vi "Real-Time-UDP.vi"() -> ()   [LabVIEW 2016]
uses:
  <vilib>/userdefined/High Color/IMAQdx.ctl
  <vilib>/FPGAPlugInAG/roboRIO/niLvFpga_Open_roboRIO.vi
  <vilib>/rvi/interface/common/dynamic/niFpgaDynamicAddResources.vi
  <vilib>/FPGAPlugInAG/Dynamic/niLvFpga_Download_Dynamic.vi
  <vilib>/FPGAPlugInAG/Dynamic/niLvFpga_Run_Dynamic.vi
  <vilib>/Utility/error.llb/Error Cluster From Error Code.vi
  <vilib>/rvi/errors/niLvFpgaAdjustHostInterfaceError.vi
  <vilib>/rvi/interface/common/niFpgaWaitOnOcc.vi
  <vilib>/vision/EDVR.llb/IMAQ ImageToEDVR 2D U32.vi
  <vilib>/FPGAPlugInAG/Dynamic/niLvFpga_Close_Dynamic.vi
  <vilib>/rvi/interface/nirviOpenFPGA/nirviOpenFPGA.xnode
  FPGA Bitfiles/ImageProcessingw_FPGATarget_ImageProcessing-_HE-F2dzEpTo.lvbitx
  <vilib>/rvi/interface/nirviMethod/nirviMethod.xnode
  <vilib>/rvi/interface/nirviReadWriteControl/nirviReadWriteControl.xnode
  <vilib>/rvi/interface/nirviCloseFPGA/nirviCloseFPGA.xnode
  <vilib>/vision/driver/NI_Vision_Acquisition_Software.lvlib
  <resource>/objmgr/imaqdx.rc
  <vilib>/rvi/interface/Simulation/niFpgaSimulationCallBeginRW.vi
  <vilib>/rvi/errors/niLvFpgaMergeErrorWithErrorCode.vi
  <vilib>/FPGAPlugInAG/Dynamic/niLvFpga_ReadFifo_Dynamic.vi
  <vilib>/FPGAPlugInAG/Dynamic/niLvFpga_ConfigureFifo_Dynamic.vi
  <vilib>/FPGAPlugInAG/Dynamic/niLvFpga_StartFifo_Dynamic.vi
  NiFpgaLv.dll
  <vilib>/FPGAPlugInAG/Dynamic/niLvFpga_WriteFifo_Dynamic.vi
panel:
  out "Image":T1(plugin-control)
  out "Error Out 2":errorcluster
  in  "Stop":bool
  in  "Maximum Pixels per Write":u32=307200
  out "dePixelCount":u32
  out "AllPixelCount":u32
  in  "Camera":T2="cam0"
  # "Overview: Demonstrates how to acquire an image from a camera using the IMAQdx API, transfer the image to a FPGA target for processing, and retrieve the processed image for display or further processing on the host.\nRequirements:\n- LabVIEW FPGA\n- Vision Acquisition Software\n- Vision Development Module\nInstructions:\n1. Select a Camera\n2. Run the VI."
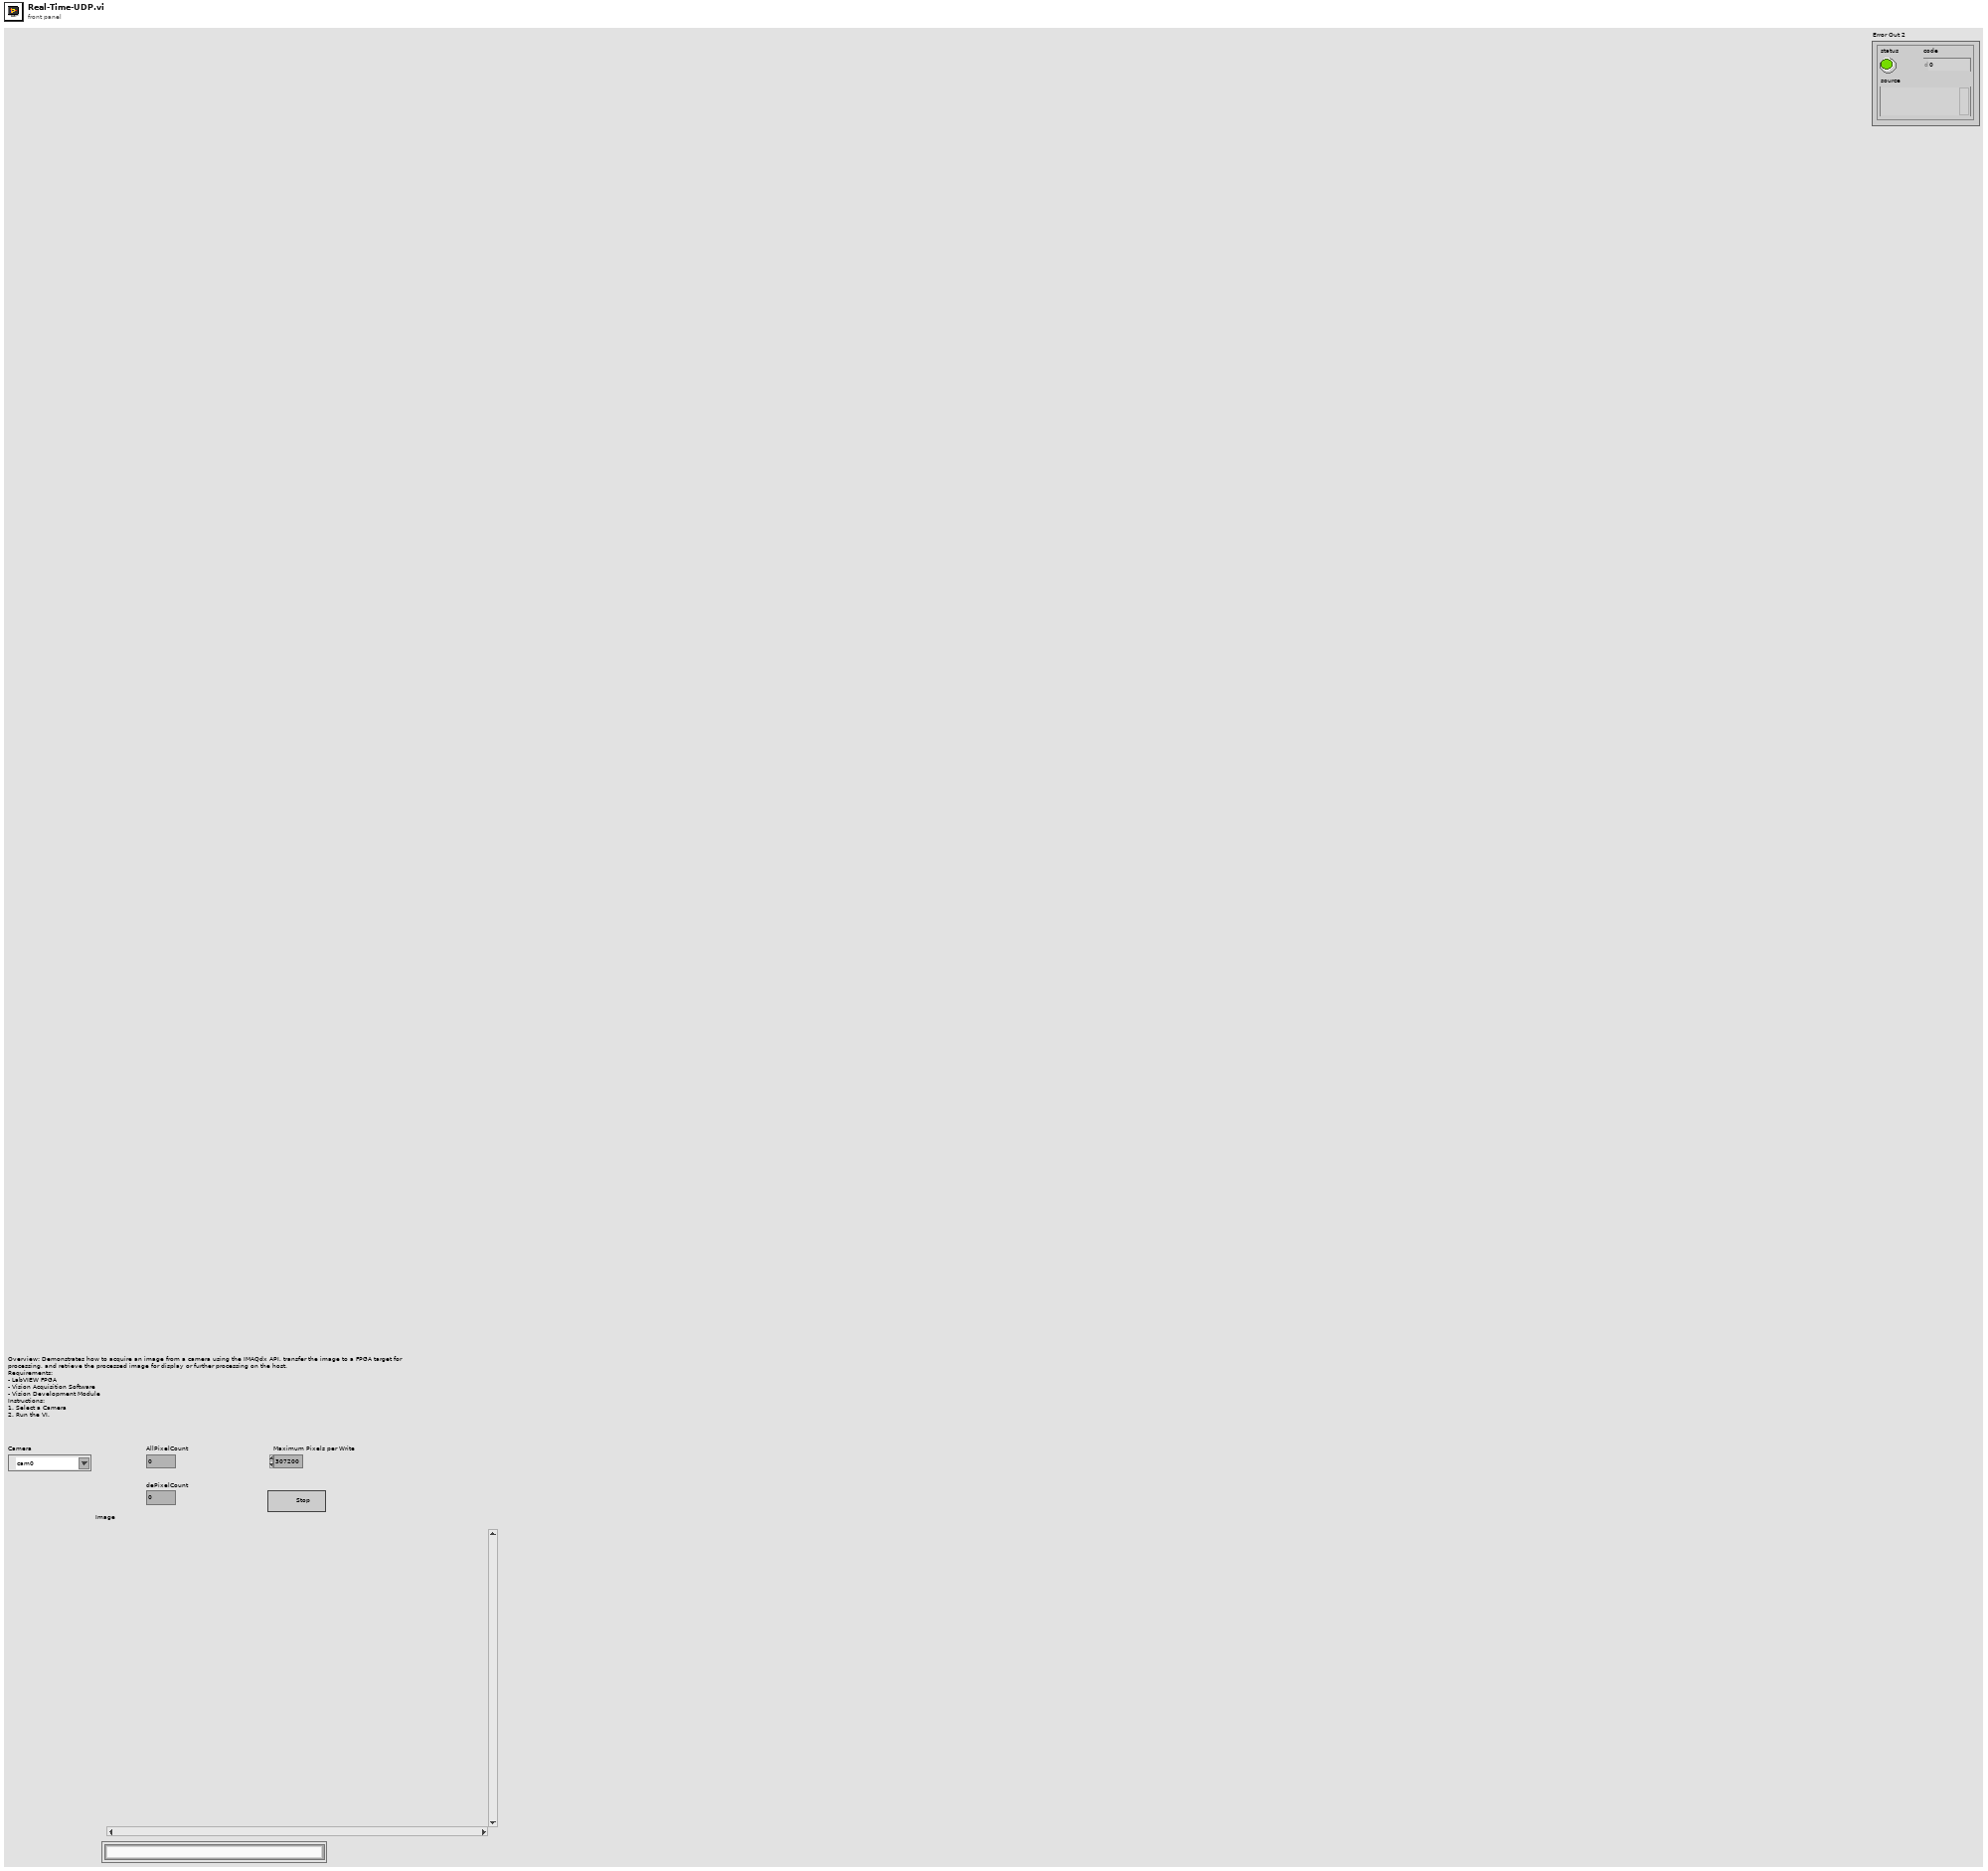
[diagram p1: front panel]
types:
  T1 = typedef "IMAQ Image.ctl" = refnum<image>
  T2 = typedef "IMAQdx.ctl" = refnum<k21>
  T3 = typedef "Image Type" = u32
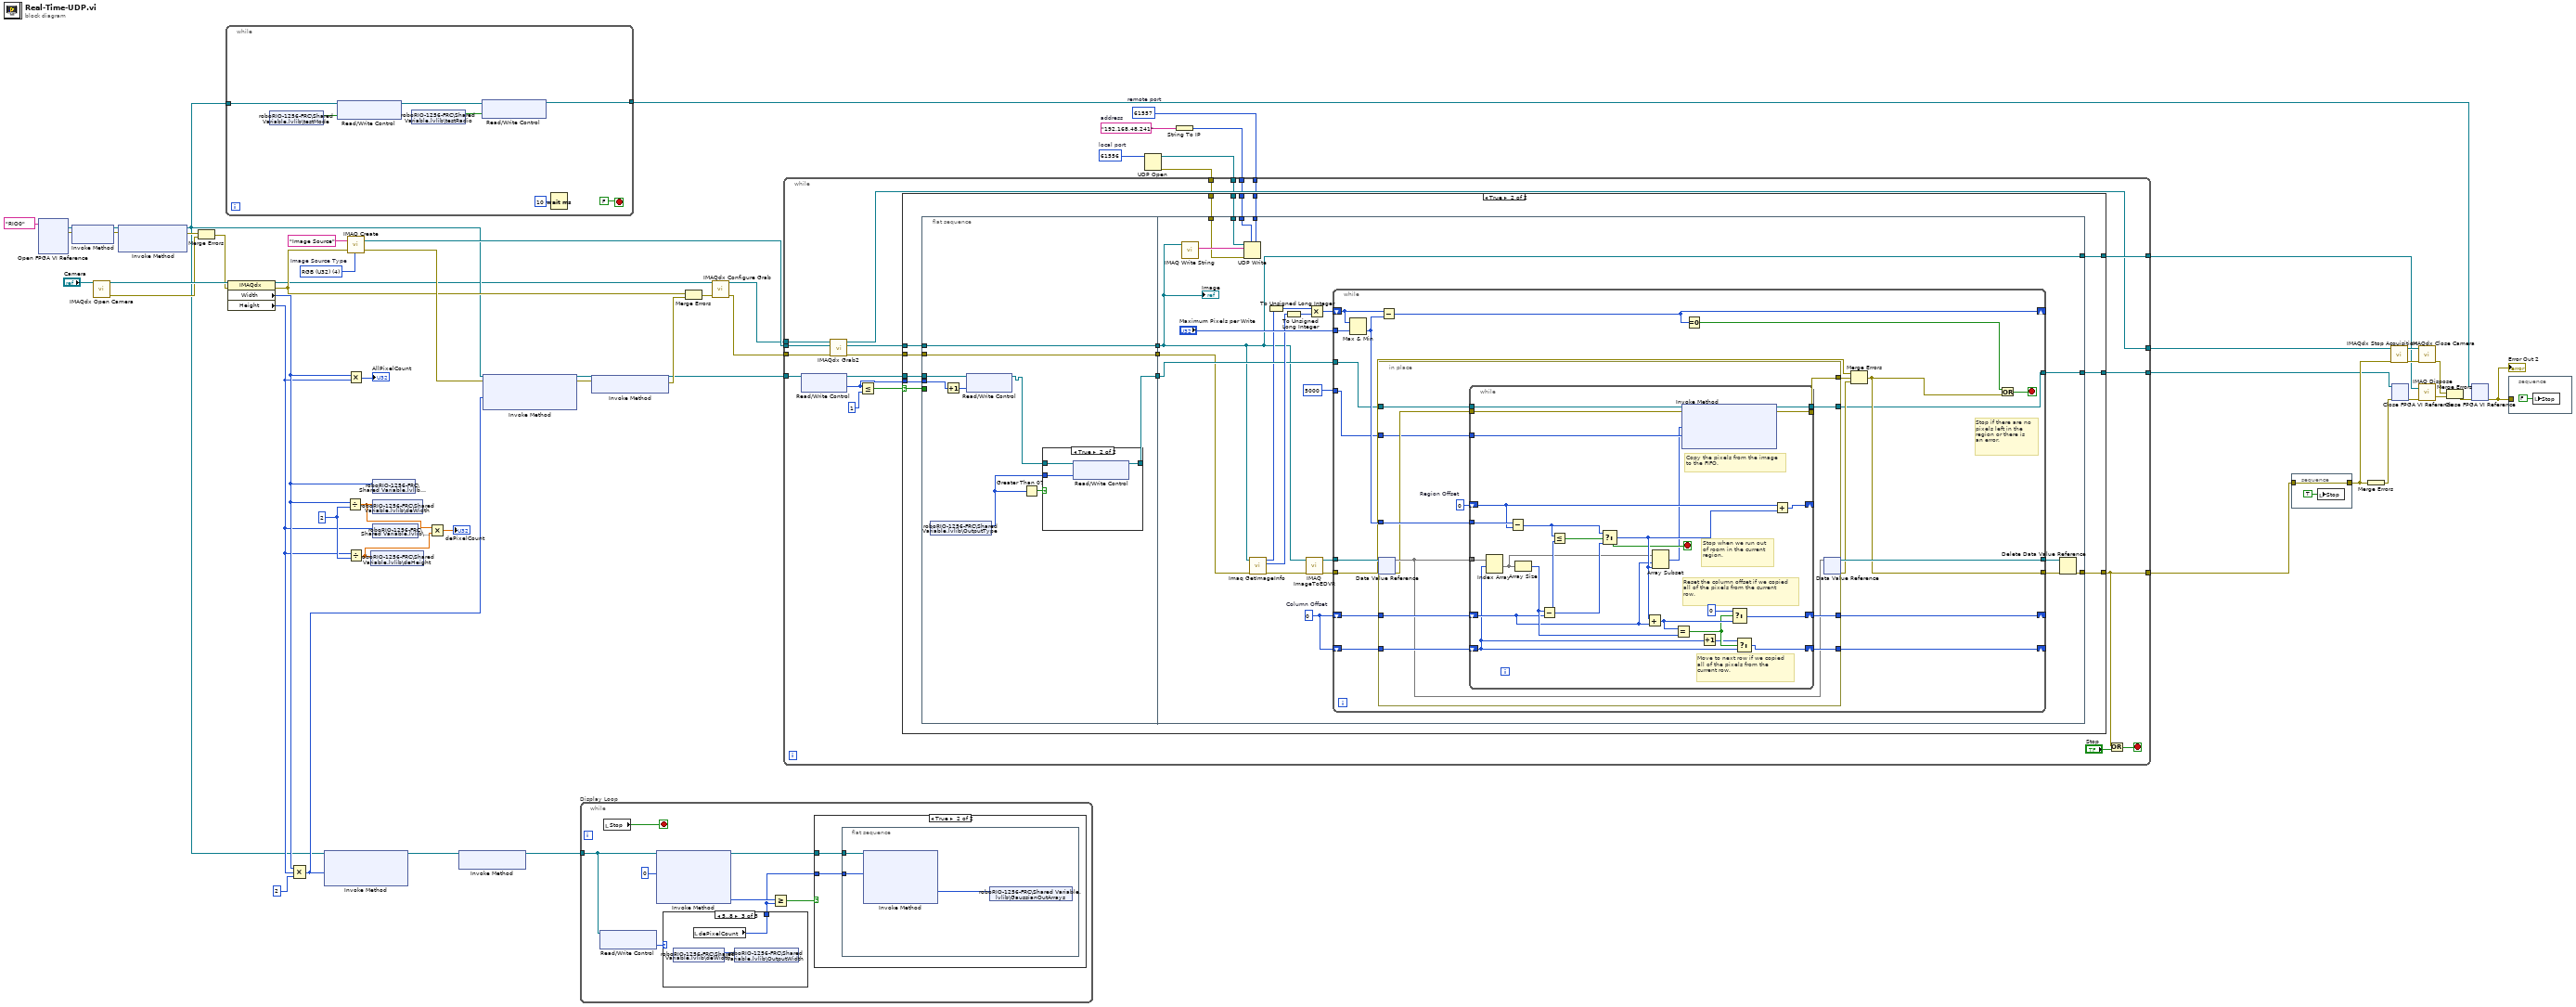
[diagram p0: block diagram]
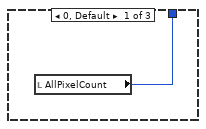
[diagram p4: hidden frame]
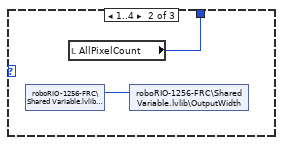
[diagram p5: hidden frame]
diagram:
  w6 = u16 61556  # local port
  w5 = "192.168.48.241"  # address
  w4 = u16 61557  # remote port
  w40 = u32 2 ("y")
  w44 = T3 4 items=["Grayscale (U8)", "Grayscale (I16)", "Grayscale (SGL)", "Complex (CSG)", "RGB (U32)", "HSL (U32)", "RGB (U64)", "Grayscale (U16)"]  # Image Source Type
  n1 = xnode "Open FPGA VI Reference"("resource name"=tag "RIO0") -> ("FPGA VI Reference Out"=w51:refnum<k20>, "error out"=w52:errorcluster)  [unwired: 1 in]
  n2 = xnode "Invoke Method"("FPGA VI Reference In"=w51, "error in"=w52) -> ("FPGA VI Reference Out"=w54:refnum<k20>, "error out"=w53:errorcluster)
  n3 = call <vilib>:"IMAQdx Open Camera.vi"("Session In"="Camera") -> ("error out"=w46:errorcluster, "Session Out"=w47:T2)  [unwired: 9 in]
  n4 = xnode "Invoke Method"("FPGA VI Reference In"=w54, "error in"=w53) -> ("FPGA VI Reference Out"=w11:refnum<k20>, "error out"=w48:errorcluster)  [unwired: 1 in]
  n5 = Merge Errors(w48, w46) -> (w45:errorcluster)
  n6 = while {
    tunnel: w11 -> [w56]
    tunnel: [w57] -> w14
    stop <- FALSE stop-if-true
    n7 = shared-variable "roboRIO-1256-FRC\\Shared Variable.lvlib\\testMode"() -> (w60:bool)  [unwired: 1 in, 1 out]
    n8 = xnode "Read/Write Control"("FPGA VI Reference In"=w56, "Mode LED Status"=w60) -> ("FPGA VI Reference Out"=w59:refnum<k20>)  [unwired: 1 in, 1 out]
    n9 = shared-variable "roboRIO-1256-FRC\\Shared Variable.lvlib\\testRadio"() -> (w58:bool)  [unwired: 1 in, 1 out]
    n10 = xnode "Read/Write Control"("FPGA VI Reference In"=w59, "Radio LED Green"=w58) -> ("FPGA VI Reference Out"=w57:refnum<k20>)  [unwired: 1 in, 1 out]
    n11 = Wait (ms)(milliseconds to wait=u32 10) -> ()  [unwired: 1 out]
  }
  n12 = property class="IMAQdx"(reference=w47, error in=w45) -> (reference out=w10:T2, error out=w29:errorcluster, "Width"=w39:u32, "Height"=w38:u32)
  n13 = Compound Arithmetic op=MULTIPLY(w39, w38, u32 2 ("value")) -> (w33:u32)
  n14 = xnode "Invoke Method"("FPGA VI Reference In"=w11, "Requested Depth"=w33) -> ("FPGA VI Reference Out"=w43:refnum<k20>)  [unwired: 1 in, 2 out]
  n15 = Divide(x=w39, y=w40) -> (x/y=w35:dbl)
  n16 = call "IMAQ Create"("Image Name"="Image Source", "Image Type"=w44, "error in (no error)"=w29) -> ("New Image"=w12:T1, "error out"=w32:errorcluster)  [unwired: 2 in]
  n17 = Multiply(x=w39, y=w38) -> (x*y=→"AllPixelCount":u32)
  n18 = Divide(x=w38, y=w40) -> (x/y=w34:dbl)
  n19 = shared-variable "roboRIO-1256-FRC\\Shared Variable.lvlib\\deHeight"(w34) -> ()  [unwired: 1 in, 1 out]
  n20 = shared-variable "roboRIO-1256-FRC\\Shared Variable.lvlib\\Width"(w39) -> ()  [unwired: 1 in, 1 out]
  n21 = shared-variable "roboRIO-1256-FRC\\Shared Variable.lvlib\\deWidth"(w35) -> ()  [unwired: 1 in, 1 out]
  n22 = shared-variable "roboRIO-1256-FRC\\Shared Variable.lvlib\\Height"(w38) -> ()  [unwired: 1 in, 1 out]
  n23 = Multiply(x=w35, y=w34) -> (x*y=→"dePixelCount":dbl)
  n24 = xnode "Invoke Method"("FPGA VI Reference In"=w43) -> ("FPGA VI Reference Out"=w42:refnum<k20>)  [unwired: 1 in, 1 out]
  n25 = xnode "Invoke Method"("FPGA VI Reference In"=w11, "error in"=w32, "Requested Depth"=w33) -> ("FPGA VI Reference Out"=w31:refnum<k20>, "error out"=w30:errorcluster)  [unwired: 1 out]
  n26 = while "Display Loop" {
    tunnel: w42 -> [w65]
    stop <- w70 stop-if-true
    n27 = xnode "Read/Write Control"("FPGA VI Reference In"=w65) -> ("getOutputType"=w64:u8)  [unwired: 1 in, 2 out]
    n28 = local read "Stop"() -> (w70:bool)
    n29 = xnode "Invoke Method"("FPGA VI Reference In"=w65, "Number of Elements"=u32 0) -> ("FPGA VI Reference Out"=w68:refnum<k20>, "Elements Remaining"=w66:u32)  [unwired: 2 in, 2 out]
    n30 = case shown="5..8" w64 {
      tunnel: [w71 w73 w75] -> w63
      frame 0, Default {
        n31 = local read "AllPixelCount"() -> (w71:u32)
      }
      frame 1..4 {
        n32 = shared-variable "roboRIO-1256-FRC\\Shared Variable.lvlib\\Width"() -> (w72:u16)  [unwired: 1 in, 1 out]
        n33 = local read "AllPixelCount"() -> (w73:u32)
        n34 = shared-variable "roboRIO-1256-FRC\\Shared Variable.lvlib\\OutputWidth"(w72) -> ()  [unwired: 1 in, 1 out]
      }
      frame 5..8 {
        n35 = shared-variable "roboRIO-1256-FRC\\Shared Variable.lvlib\\deWidth"() -> (w74:u16)  [unwired: 1 in, 1 out]
        n36 = local read "dePixelCount"() -> (w75:u32)
        n37 = shared-variable "roboRIO-1256-FRC\\Shared Variable.lvlib\\OutputWidth"(w74) -> ()  [unwired: 1 in, 1 out]
      }
    }
    n38 = Greater Or Equal?(x=w66, y=w63) -> (x >= y?=w67:bool)
    n39 = case shown="True" w67 {
      tunnel: w68 -> [_ w77]
      tunnel: w63 -> [_ w76]
      frame False {
      }
      frame True {
        n40 = flat-sequence {
          tunnel: w77 -> [w80]
          tunnel: w76 -> [w79]
          frame #0 {
            n41 = xnode "Invoke Method"("FPGA VI Reference In"=w80, "Number of Elements"=w79) -> ("Data"=w78:u8[])  [unwired: 2 in, 3 out]
            n42 = shared-variable "roboRIO-1256-FRC\\Shared Variable.lvlib\\GaussianOutArrays"(w78) -> ()  [unwired: 1 in, 1 out]
          }
        }
      }
    }
  }
  n43 = xnode "Invoke Method"("FPGA VI Reference In"=w31, "error in"=w30) -> ("FPGA VI Reference Out"=w13:refnum<k20>, "error out"=w28:errorcluster)
  n44 = Merge Errors(w29, w28) -> (w9:errorcluster)
  n45 = call <vilib>:"IMAQdx Configure Grab.vi"("error in"=w9, "Session In"=w10) -> ("error out"=w7:errorcluster, "Session Out"=w8:T2)  [unwired: 8 in]
  n46 = UDP Open(11:w6) -> (port=w2:refnum<k16>, 0:w1:errorcluster)  [unwired: 4 in, 1 out]
  n47 = String To IP(1:w5) -> (0:w3:u32)
  n48 = while {
    tunnel: [w95] -> w18
    tunnel: w8 -> [w92]
    tunnel: w12 -> [w91]
    tunnel: w7 -> [w90]
    tunnel: w13 -> [w86]
    tunnel: [w98] -> w16
    tunnel: [w97] -> w17
    tunnel: [w96] -> w15
    tunnel: w4 -> [w84]
    tunnel: w3 -> [w83]
    tunnel: w2 -> [w82]
    tunnel: w1 -> [w81]
    stop <- w99 stop-if-true
    n49 = xnode "Read/Write Control"("FPGA VI Reference In"=w86) -> ("FPGA VI Reference Out"=w88:refnum<k20>, "picRemains"=w87:u8)  [unwired: 1 in, 1 out]
    n50 = call <vilib>:"IMAQdx Grab2.vi"("error in"=w90, "Image In"=w91, "Session In"=w92) -> ("error out"=w93:errorcluster, "Image Out"=w94:T1, "Session Out"=w95:T2)  [unwired: 5 in, 1 out]
    n51 = Less Or Equal?(x=w87, y=u8 1) -> (x <= y?=w85:bool)
    n52 = case shown="True" w85 {
      selector: w85 -> [_ w110]
      tunnel: w88 -> [w102 w118]
      tunnel: w94 -> [w103 w114]
      tunnel: [w101 w117] -> w98
      tunnel: w93 -> [w101 w116]
      tunnel: [w102 w115] -> w97
      tunnel: [w103 w109] -> w96
      tunnel: w87 -> [_ w108]
      tunnel: w84 -> [_ w107]
      tunnel: w83 -> [_ w106]
      tunnel: w82 -> [_ w105]
      tunnel: w81 -> [_ w104]
      frame False {
      }
      frame True {
        n53 = flat-sequence {
          tunnel: w114 -> [w126]
          tunnel: w116 -> [w127]
          tunnel: w118 -> [w122]
          tunnel: [w125] -> w113
          tunnel: [w127] -> w112
          tunnel: [w126] -> w111
          tunnel: w110 -> [_]
          tunnel: w108 -> [w119]
          tunnel: [w140] -> w117
          tunnel: [w138] -> w115
          tunnel: w113 -> [w142]
          tunnel: w112 -> [w139]
          tunnel: w111 -> [w132]
          tunnel: [w132] -> w109
          tunnel: w107 -> [w136]
          tunnel: w106 -> [w135]
          tunnel: w105 -> [w134]
          tunnel: w104 -> [w133]
          frame #0 {
            n54 = shared-variable "roboRIO-1256-FRC\\Shared Variable.lvlib\\OutputType"() -> (w123:u8)  [unwired: 1 in, 1 out]
            n55 = Increment(x=w119) -> (x+1=w120:u8)
            n56 = xnode "Read/Write Control"("FPGA VI Reference In"=w122, "picRemains"=w120) -> ("FPGA VI Reference Out"=w121:refnum<k20>)  [unwired: 1 in, 1 out]
            n57 = Greater Than 0?(x=w123) -> (x > 0?=w124:bool)
            n58 = case shown="True" w124 {
              tunnel: w121 -> [w128 w131]
              tunnel: [w128 w130] -> w125
              tunnel: w123 -> [_ w129]
              frame False {
              }
              frame True {
                n59 = xnode "Read/Write Control"("FPGA VI Reference In"=w131, "setOutputType"=w129) -> ("FPGA VI Reference Out"=w130:refnum<k20>)  [unwired: 1 in, 1 out]
              }
            }
          }
          frame #1 {
            w144 = u32 0  # Column Offset
            n60 = call-poly "IMAQ Write String"("Image"=w132) -> ("FileString"=w137:string)  [unwired: 8 in, 2 out]
            n61 = UDP Write(address=w135, port or service name=w136, connection ID=w134, data in=w137, 8:w133) -> ()  [unwired: 1 in, 2 out]
            n62 = call "Imaq GetImageInfo"("error in (no error)"=w139, "Image"=w132) -> ("error out"=w150:errorcluster, "Y Resolution"=w151:i32, "X Resolution"=w141:i32)  [unwired: 2 in, 5 out]
            n63 = To Unsigned Long Integer(number=w141) -> (unsigned 32bit integer=w153:u32)
            n64 = To Unsigned Long Integer(number=w151) -> (unsigned 32bit integer=w154:u32)
            n65 = call-poly <vilib>:"IMAQ ImageToEDVR.vi"("error out"=w150, "Image"=w132) -> ("error out"=w148:errorcluster, "EDVR 2D U32"=w149:refnum<data-value>)  [unwired: 7 in, 1 out]
            n66 = Multiply(x=w153, y=w154) -> (x*y=w145:u32)
            n67 = while {
              shift-right: [w167] -> _
              shift-left: w145 -> [w164]
              tunnel: w149 -> [w173]
              shift-right: [w169] -> _
              shift-left: w144 -> [w171]
              shift-right: [w172] -> _
              shift-left: w144 -> [w170]
              tunnel: w142 -> [w157]
              tunnel: [w168] -> w147
              tunnel: [w159] -> w146
              tunnel: "Maximum Pixels per Write" -> [w163]
              tunnel: 5000 ("Write Timeout (ms)") -> [w156]
              tunnel: w148 -> [w158]
              tunnel: [w155] -> w138
              stop <- w166 stop-if-true
              # "Stop if there are no\npixels left in the \nregion or there is\nan error."
              n68 = Max & Min(x=w164, y=w163) -> (min(x,y)=w162:u32)  [unwired: 1 out]
              n69 = in-place {
                in-place-border: w162 -> [w183]
                in-place-border: [w185] -> w172
                in-place-border: w171 -> [w182]
                in-place-border: w170 -> [w180]
                in-place-border: [w181] -> w169
                in-place-border: [w176] -> w161
                in-place-border: w157 -> [w178]
                in-place-border: w156 -> [w175]
                in-place-border: [w174] -> w155
                w184 = u32 0  # Region Offset
                n70 = in-place-dvr #1(w173) -> (w179:u32[][], w177:errorcluster)
                n71 = while {
                  tunnel: w179 -> [w195]
                  shift-right: [w207] -> _
                  shift-left: w184 -> [w206]
                  tunnel: w183 -> [w209]
                  shift-right: [w200] -> w181
                  shift-left: w182 -> [w196]
                  shift-right: [w197] -> w185
                  shift-left: w180 -> [w193]
                  tunnel: w178 -> [w191]
                  tunnel: w177 -> [w190]
                  tunnel: [w189] -> w176
                  tunnel: w175 -> [w188]
                  tunnel: [w186] -> w174
                  stop <- w192 stop-if-true
                  # "Copy the pixels from the image\nto the FIFO."
                  # "Stop when we run out\nof room in the current\nregion."
                  # "Reset the column offset if we copied\nall of the pixels from the current\nrow."
                  # "Move to next row if we copied\nall of the pixels from the\ncurrent row."
                  n72 = Index Array(array=w195, index (row)=w193) -> (element=w194:u32[])  [unwired: 1 in]
                  n73 = Subtract(x=w209, y=w206) -> (x-y=w208:u32)
                  n74 = Array Size(array=w194) -> (size(s)=w205:i32)
                  n75 = Subtract(x=w205, y=w196) -> (x-y=w203:u32)
                  n76 = Less Or Equal?(x=w208, y=w203) -> (x <= y?=w192:bool)
                  n77 = Select(t=w208, s=w192, f=w203) -> (s? t:f=w204:u32)
                  n78 = Add(x=w204, y=w196) -> (x+y=w201:u32)
                  n79 = Array Subset(array=w194, index=w196, length=w204) -> (w187:u32[])
                  n80 = Equal?(x=w201, y=w205) -> (x = y?=w199:bool)
                  n81 = xnode "Invoke Method"("FPGA VI Reference In"=w191, "error in"=w190, "Data"=w187, "Timeout (ms)"=w188) -> ("FPGA VI Reference Out"=w186:refnum<k20>, "error out"=w189:errorcluster)  [unwired: 1 out]
                  n82 = Increment(x=w193) -> (x+1=w198:u32)
                  n83 = Select(t=u32 0 ("Elements In Region"), s=w199, f=w201) -> (s? t:f=w200:u32)
                  n84 = Select(t=w198, s=w199, f=w193) -> (s? t:f=w197:u32)
                  n85 = Add(x=w206, y=w204) -> (x+y=w207:u32)
                }
                n86 = in-place-dvr #1(w179) -> (w168:refnum<data-value>, w160:errorcluster)
              }
              n87 = Subtract(x=w164, y=w162) -> (x-y=w167:u32)
              n88 = Equal To 0?(x=w167) -> (x = 0?=w165:bool)
              n89 = Merge Errors(w158, w161, w160) -> (w159:errorcluster)
              n90 = Or(x=w165, y=w159) -> (x .or. y?=w166:bool)
            }
            n91 = Delete Data Value Reference(data value reference=w147, error in=w146) -> (error out=w140:errorcluster)  [unwired: 1 out]
            "Image" <- w132
          }
        }
      }
    }
    n92 = Or(x=w98, y="Stop") -> (x .or. y?=w99:bool)
  }
  n93 = stacked-sequence {
    tunnel: w16 -> [w210]
    tunnel: [w210] -> w19
    frame #0 {
      n94 = local write "Stop"(TRUE ("Stop")) -> ()
    }
  }
  n95 = Merge Errors(w19) -> (w20:errorcluster)
  n96 = call <vilib>:"IMAQdx Stop Acquisition.vi"("error in"=w19, "Session In"=w18) -> ("error out"=w24:errorcluster, "Session Out"=w25:T2)  [unwired: 8 in]
  n97 = xnode "Close FPGA VI Reference"("FPGA VI Reference In"=w17, "error in"=w20) -> ("error out"=w27:errorcluster)
  n98 = call <vilib>:"IMAQdx Close Camera.vi"("error in"=w24, "Session In"=w25) -> ("error out"=w23:errorcluster)  [unwired: 9 in]
  n99 = call "IMAQ Dispose"("Image"=w15, "error in (no error)"=w27) -> ("error out"=w26:errorcluster)  [unwired: 4 in]
  n100 = Merge Errors(w23, w26) -> (w22:errorcluster)
  n101 = xnode "Close FPGA VI Reference"("FPGA VI Reference In"=w14, "error in"=w22) -> ("error out"=w21:errorcluster)
  "Error Out 2" <- w21
  n102 = stacked-sequence {
    tunnel: w21 -> [_]
    frame #0 {
      n103 = local write "Stop"(FALSE ("Stop")) -> ()
    }
  }
